vi "log_fifo_fxp_mask.vi"(4 "Timeout(ticks)":i32=500, 6 "Log-Channel_select":bool[](array[boolean])=[TRUE, TRUE, TRUE, TRUE, FALSE, FALSE], 8 "FIFO In":refnum<k21>="FPGA_TO_HOST_FXP", 11 "input-data":fxp<+/-,16,5>[](array[numeric])=[0.0, 0.0, 0.0, 0.0, 0.0]) -> (3 "logging-timeout?":bool)   [LabVIEW 2017]
uses:
  <vilib>/rvi/DataTransferAndStorage/Container/Common/niFpgaContainerExecOnDevCompGetState.vi
  <vilib>/rvi/Emulation/niFpgaEmulationIsFPGAContextNoSignature.vi
  <vilib>/rvi/Emulation/niFpgaSctlEmulationGetInTimedLoop.vi
  <vilib>/rvi/errors/niFpgaSetErrorForExecOnDevCompSimple.vi
  <vilib>/rvi/eio/common/nirviEmuReportErrorAndStop.vi
  <vilib>/rvi/DataTransferAndStorage/Container/Common/niFpgaContainerGetUniqueNameForEmu.vi
  <vilib>/rvi/FIFO/Fifo_Resource/nirvififoEmulationSetSize.vi
  <vilib>/rvi/FIFO/Fifo_Resource/nirviFifoEmulationQueueMgr.vi
  <instcachedir>/0/nirviFifoEmulationQueueMgr_E5CAEC123FF24DC58D834DCA3CDAA9B5.lvgen/nirviFifoEmulationQueueMgr_E5CAEC123FF24DC58D834DCA3CDAA9B5_001.vi
  <vilib>/rvi/FIFO/Fifo_Resource/nirvififoEmulationDetermineInputValidOut.vi
  <vilib>/rvi/FIFO/Fifo_Resource/nirvififoEmulationCreateLock.vi
  <vilib>/rvi/Emulation/niFpgaProcessEmulError.vi
  <vilib>/rvi/FIFO/Fifo_Resource/nirvififoEmulationObtainLock.vi
  <vilib>/rvi/FIFO/Fifo_Resource/nirvififoEmulationReleaseLock.vi
  <vilib>/rvi/occurrence/nirviWaitOnOccurrenceBase.vi
  <vilib>/rvi/errors/nirviReportUnexpectedCaseInternalError.vi
  <vilib>/rvi/errors/nirviReportUnexpectedCaseInternalError (U32).vi
  <vilib>/Utility/error.llb/Clear Errors.vi
  <vilib>/rvi/interface/RandomDataEmulation/niFpgaRandomDataHandleErrors.vi
  <vilib>/rvi/DataTransferAndStorage/Container/XNode/niFpgaContainer.xnode
  <vilib>/rvi/FIFO/Fifo_Resource/niFpgaFifoEmulationRefIn.vi
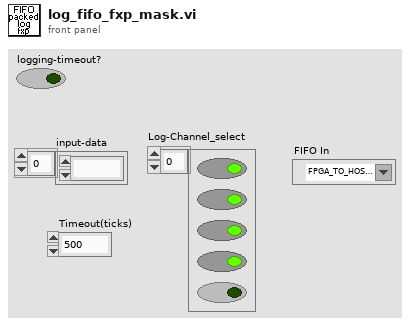
[diagram p1: front panel]
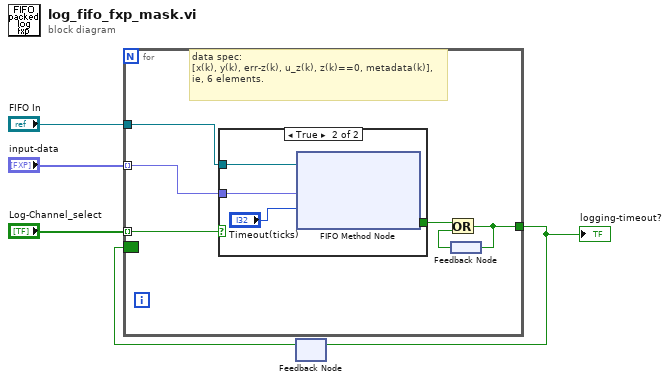
[diagram p0: block diagram]
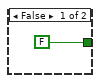
[diagram p2: hidden frame]
diagram:
  n1 = feedback #1() -> (w3:bool)  [unwired: 1 in]
  n2 = for {
    tunnel: "input-data" -> [w11] mode=indexing
    tunnel: [w8] -> w5
    border: w3 -> [_]
    tunnel: "FIFO In" -> [w7]
    tunnel: "Log-Channel_select" -> [w6] mode=indexing
    # "data spec:\n[x(k), y(k), err-z(k), u_z(k), z(k)==0, metadata(k)],\nie, 6 elements."
    n3 = case shown="True" w6 {
      tunnel: w11 -> [_ w16]
      tunnel: [FALSE ("Timed Out?") w15] -> w10
      tunnel: w7 -> [_ w14]
      frame False {
      }
      frame True {
        n4 = xnode ("FIFO Method Node")("Element"=w16, "Timeout"="Timeout(ticks)", "FIFO In"=w14) -> ("Timed Out?"=w15:bool)  [unwired: 1 out]
      }
    }
    n5 = feedback #2() -> (w9:bool)
    n6 = Or(x=w10, y=w9) -> (x .or. y?=w8:bool)
    n7 = feedback-in #2(w8) -> ()
  }
  "logging-timeout?" <- w5
  n8 = feedback-in #1(w5) -> ()
